vi "Ends_With.vi"(2 "Ending":string, 3 "string":string) -> (0 "Ending To Large?":bool, 1 "Ends WIth?":bool)   [LabVIEW 2016]
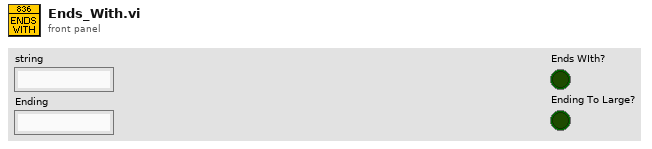
[diagram p1: front panel]
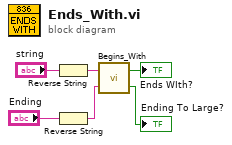
[diagram p0: block diagram]
diagram:
  n1 = Reverse String(1:"string") -> (0:w4:string)
  n2 = Reverse String(1:"Ending") -> (0:w3:string)
  n3 = call <userlib>:"Begins_With.vi"("Beginning"=w3, "String"=w4) -> ("Beginning To Large?"=→"Ending To Large?":bool, "Begins With?"=→"Ends WIth?":bool)
